vi "UniqueNameCheck.vi"(9 "Names in use":string[](array[string]), 10 "Device Name":string) -> (1 "Names in use out":string[](array[string]), 2 "Unique name":string)   [LabVIEW 2013]
doc: "Check new name against list of reserved name. If on reserved list, prompt for new name with dialog. Add new name to list of reserved names."
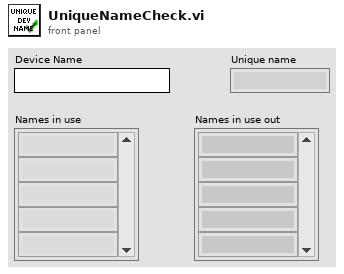
[diagram p1: front panel]
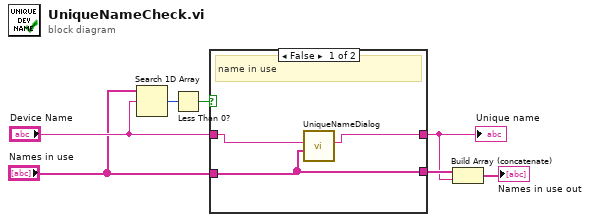
[diagram p0: block diagram]
diagram:
  n1 = Search 1D Array(1D array="Names in use", element="Device Name") -> (index of element=w7:i32)  [unwired: 1 in]
  n2 = Less Than 0?(x=w7) -> (x < 0?=w6:bool)
  n3 = case shown="False" w6 {
    tunnel: "Device Name" -> [w10 w12]
    tunnel: [w9 w12] -> w2
    tunnel: "Names in use" -> [w8 w11]
    tunnel: [w8 w11] -> w3
    frame False {
      # "name in use"
      n4 = call "UniqueNameDialog.vi"("Names in use"=w8, "Device Name"=w10) -> ("Unique name"=w9:string)  [unwired: 9 in]
    }
    frame True {
      # "unique."
    }
  }
  "Unique name" <- w2
  n5 = Build Array (concatenate)(w3, w2) -> (→"Names in use out":string[])
